vi "Set daemon termination flag.vi"(6 "Message":string, 8 "error in (no error)":errorcluster, 9 "Reason URI":string, 10 "Reason":T1, 11 "WAMP Client (in)":refnum<class "WAMP Client.lvclass">) -> (0 "error out":errorcluster, 3 "WAMP Client (out)":refnum<class "WAMP Client.lvclass">)   [LabVIEW 2020, in "wamplv.lvlib" / "WAMP Client.lvclass"]
uses:
  WAMP Client.lvclass
  WAMP Client.lvclass/WAMP Client.ctl
  TypeDef/Termination Reason Enum.ctl
  API/TypeDefs/Termination Reason.ctl
  TypeDef/Termination Request.ctl
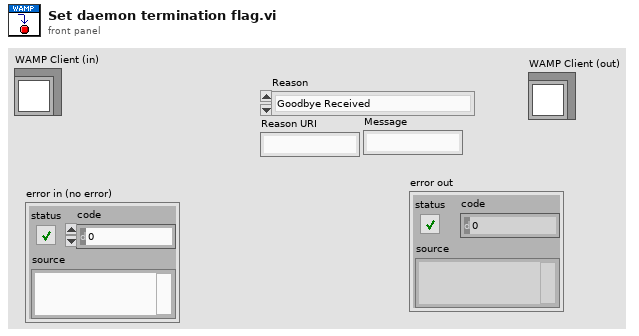
[diagram p1: front panel]
types:
  T1 = typedef "wamplv.lvlib/WAMP Client.lvclass/Termination Reason Enum.ctl" = enum16{"Goodbye Received", "Abort Received", "Send Goodbye", "Send Abort", "Read Loop Failure", "Write Loop Failure", "Message Loop Failure"}
  T2 = typedef "wamplv.lvlib/WAMP Client.lvclass/Termination Reason.ctl" = cluster{"Reason":T1, "Reason URI":string, "Message":string}
  T3 = typedef "wamplv.lvlib/WAMP Client.lvclass/Termination Request.ctl" = cluster{"Terminate?":bool, "Termination Reason":T2}
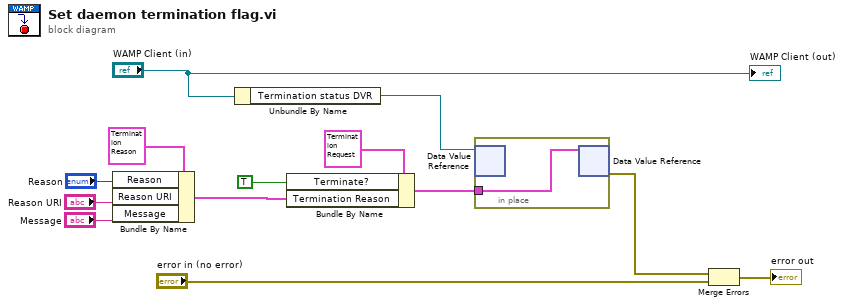
[diagram p0: block diagram]
diagram:
  n1 = Bundle By Name(cluster=T2 {"Reason"=enum."Goodbye Received", "Reason URI"="wamp.error.protocol_violation", "Message"=""} ("Termination Reason"), "Reason"="Reason", "Reason URI"="Reason URI", "Message"="Message") -> (w6:T2)
  n2 = Unbundle By Name("WAMP Client (in)") -> ("Termination status DVR"=w9:refnum<data-value>)
  n3 = Bundle By Name(cluster=T3 {"Terminate?"=FALSE, "Termination Reason"={"Reason"=enum."Goodbye Received", "Reason URI"="wamp.error.protocol_violation", "Message"=""}} ("Daemon Termination Request"), "Terminate?"=TRUE, "Termination Reason"=w6) -> (w1:T3)
  n4 = in-place {
    in-place-border: w1 -> [w14]
    n5 = in-place-dvr #1(w9) -> ()  [unwired: 2 out]
    n6 = in-place-dvr #1(w14) -> (w12:errorcluster)  [unwired: 1 out]
  }
  n7 = Merge Errors(w12, "error in (no error)") -> (→"error out":errorcluster)
  "WAMP Client (out)" <- "WAMP Client (in)"
